vi "Cash Karp Function.vi"(6 "X":dbl[](array[numeric]) format="%.2f", 7 "time":dbl format="%.2f", 8 "result":dbl[][](array[numeric]) format="%.2f", 9 "table":i32[][][](array[numeric]), 10 "X":string[](array[string])=["x1", "x2"], 11 "time":string="t") -> (3 "F(X,time)":dbl[](array[numeric]) format="%.2f")   [LabVIEW 2020, in "NI_Gmath.lvlib"]
uses:
  <vilib>/gmath/NI_Gmath.lvlib
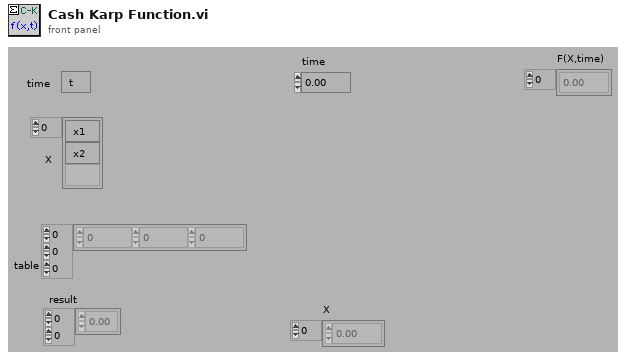
[diagram p1: front panel]
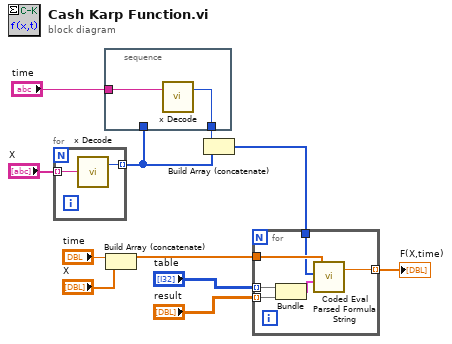
[diagram p0: block diagram]
diagram:
  n1 = for {
    tunnel: "X" -> [w13] mode=indexing
    tunnel: [w12] -> w5 mode=indexing
    n2 = call <vilib>:"x Decode.vi"("x string"=w13) -> ("number"=w12:i32)  [unwired: 1 in, 1 out]
  }
  n3 = stacked-sequence {
    tunnel: [w15] -> w9
    tunnel: w5 -> [_]
    tunnel: "time" -> [w14]
    frame #0 {
      n4 = call <vilib>:"x Decode.vi"("x string"=w14) -> ("number"=w15:i32)  [unwired: 1 in, 1 out]
    }
  }
  n5 = Build Array (concatenate)("time", "X") -> (w10:dbl[])
  n6 = Build Array (concatenate)(w9, w5) -> (w8:i32[])
  n7 = for {
    tunnel: w8 -> [w19]
    tunnel: w10 -> [w20]
    tunnel: [w21] -> w7 mode=indexing
    tunnel: "result" -> [w17] mode=indexing
    tunnel: "table" -> [w18] mode=indexing
    n8 = Bundle("table"=w18, "result"=w17) -> (w16:cluster{"table":i32[][], "result":dbl[]})  [unwired: 1 in]
    n9 = call <vilib>:"Coded Eval Parsed Formula String.vi"("Parsed Formula"=w16, "Variables"=w19, "X Values"=w20) -> ("y value"=w21:dbl)  [unwired: 1 in, 1 out]
  }
  "F(X,time)" <- w7
